vi "workspace.display_name.vi"(8 "error in":errorcluster, 11 "Workspace in":refnum<class "Workspace.lvclass">) -> (0 "error out":errorcluster, 3 "Workspace out":refnum<class "Workspace.lvclass">)   [LabVIEW 2020, in "Workspace.lvclass"]
doc: "Returns the workspace's display name."
uses:
  Workspace.lvclass
  Workspace.lvclass/Workspace.ctl
  client.lvlib
panel:
  out "out_needed out":u32
  out "display name":string
  out "is_present out":bool
  in  "out_needed":u32
  in  "cap":u32
  in  "buf":string
  in  "is_present":bool
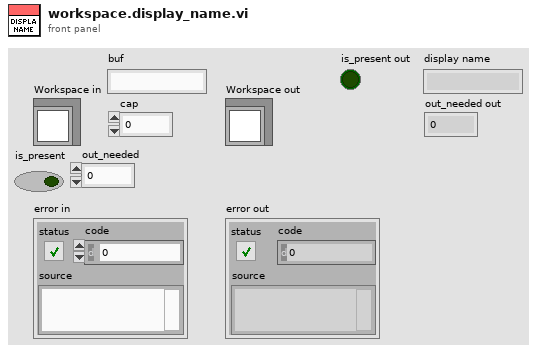
[diagram p1: front panel]
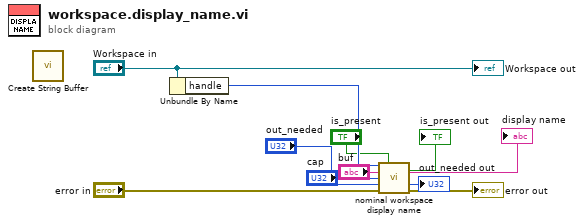
[diagram p0: block diagram]
diagram:
  n1 = call "Create String Buffer.vi"() -> ()  [unwired: 9 in, 3 out]
  n2 = Unbundle By Name("Workspace in") -> ("handle"=w9:i32)
  n3 = call "nominal workspace display name.vi"("workspace"=w9, "is_present"="is_present", "buf"="buf", "cap"="cap", "out_needed"="out_needed", "error in (no error)"="error in") -> ("is_present out"=→"is_present out":bool, "buf out"=→"display name":string, "out_needed out"=→"out_needed out":u32, "error out"=→"error out":errorcluster)  [unwired: 5 in, 1 out]
  "Workspace out" <- "Workspace in"
